vi "Get Picture.vi"(8 "error in (no error)":errorcluster, 11 "Electronic Parts in":refnum<class "Electronic Parts.lvclass">) -> (0 "error out":errorcluster, 2 "Picture":picture, 3 "Electronic Parts out":refnum<class "Electronic Parts.lvclass">)   [LabVIEW 2020, in "Electronic Parts.lvclass"]
uses:
  Electronic Parts.lvclass
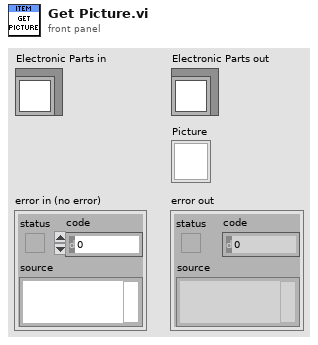
[diagram p1: front panel]
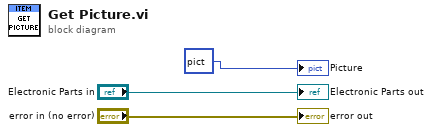
[diagram p0: block diagram]
diagram:
  "error out" <- "error in (no error)"
  "Electronic Parts out" <- "Electronic Parts in"
  "Picture" <- picture bytes[3230] ("new picture")
